vi "Close Device Driver.vi"(8 "error in (no error)":errorcluster, 11 "IVI_DMM in":refnum<class "IVI_DMM.lvclass">) -> (0 "error out":errorcluster, 3 "IVI_DMM out":refnum<class "IVI_DMM.lvclass">)   [LabVIEW 2013, in "IVI_DMM.lvlib" / "IVI_DMM.lvclass"]
doc: "Close device driver connection."
uses:
  IVI_DMM.lvclass
  Base/CS++DMM/CS++DMM.lvclass
  IVI_DMM.lvclass/IVI_DMM.ctl
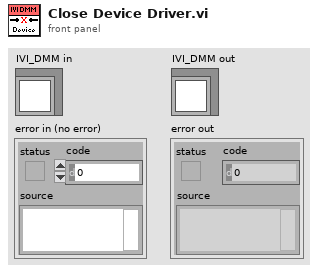
[diagram p1: front panel]
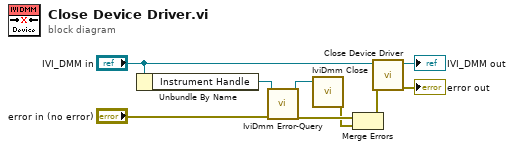
[diagram p0: block diagram]
diagram:
  n1 = Unbundle By Name("IVI_DMM in") -> ("Instrument Handle"=w6:refnum<k15>)
  n2 = call <vilib>:"IviDmm Error-Query.vi"("error in (no error)"="error in (no error)", "instrument handle"=w6) -> ("error out"=w3:errorcluster, "instrument handle out"=w5:refnum<k15>)  [unwired: 6 in, 2 out]
  n3 = call <vilib>:"IviDmm Close.vi"("instrument handle"=w5) -> ("error out"=w2:errorcluster)  [unwired: 10 in]
  n4 = Merge Errors(w3, w2) -> (w1:errorcluster)
  n5 = call-parent "Close Device Driver.vi"("error in (no error)"=w1, "CS++DMM in"="IVI_DMM in") -> ("error out"=→"error out":errorcluster, "CS++DMM out"=→"IVI_DMM out":refnum<class "IVI_DMM.lvclass">)  [unwired: 8 in]
